vi "Sequencer Do.vi"(8 "error in (no error)":errorcluster, 10 "Sequencer in":refnum<class "Sequencer.lvclass">, 11 "Terminate Sequencer Msg":refnum<class "Terminate Sequencer Msg.lvclass">) -> (0 "error out":errorcluster, 2 "Sequencer out":refnum<class "Sequencer.lvclass">)   [LabVIEW 2020, in "Sequencer.lvlib" / "Terminate Sequencer Msg.lvclass"]
doc: "The action the Sequencer Msg performs in the Sequencers Recieve Message method.\nThe default implementation forwards the message to hte Sequencer Core."
uses:
  Terminate Sequencer Msg.lvclass
  Sequencer/Sequencer.lvclass
  C:/Current projects/WS/PPL/HDH.Actor Framework.Core.Actor.lvlibp/1abvi3w/vi.lib/ActorFramework/Actor/Actor.lvclass
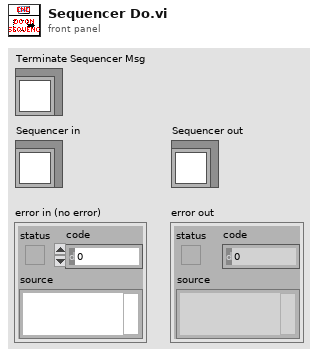
[diagram p1: front panel]
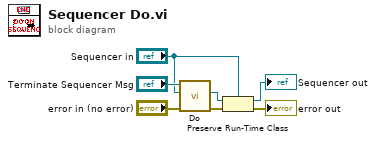
[diagram p0: block diagram]
diagram:
  n1 = call-dynamic "Do.vi"("error in (no error)"="error in (no error)", "Actor in"="Sequencer in", "Terminate Sequencer Msg"="Terminate Sequencer Msg") -> ("error out"=w2:errorcluster, "Actor out"=w6:refnum<class "Actor.lvclass">)  [unwired: 7 in]
  n2 = Preserve Run-Time Class(object in=w6, error in=w2, 2:"Sequencer in") -> (object out=→"Sequencer out":refnum<class "Sequencer.lvclass">, error out=→"error out":errorcluster)
